vi "Create and Enqueue Self Launch.vi"(8 "error in (no error)":errorcluster) -> (0 "error out":errorcluster, 3 "Internal-Launch":refnum<event-registration>)   [LabVIEW 2018, in "Scripting.lvlib" / "Actor.lvlib" / "Actor.lvclass"]
uses:
  Actor.lvclass
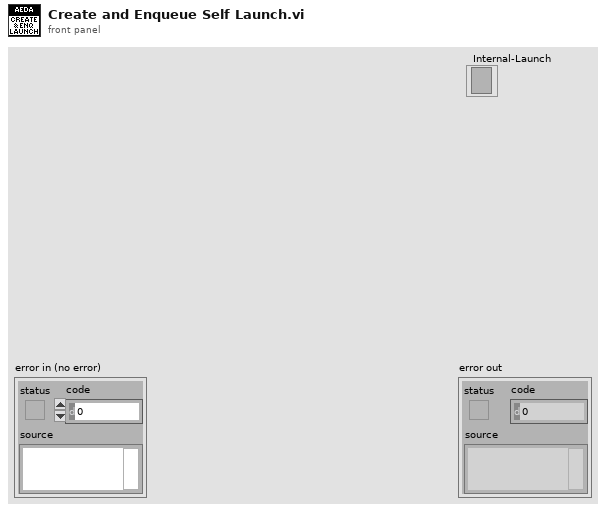
[diagram p1: front panel]
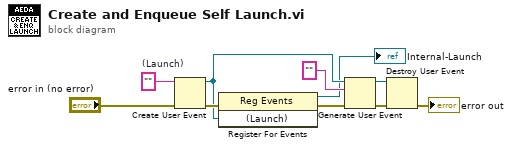
[diagram p0: block diagram]
diagram:
  w3 = ""  # (Launch)
  n1 = Create User Event(user event datatype=w3, error in="error in (no error)") -> (user event=w7:refnum<user-event>, error out=w10:errorcluster)
  n2 = register-events(error in=w10, w7) -> (reference out=→"Internal-Launch":refnum<event-registration>, error out=w8:errorcluster)  [unwired: 1 in]
  n3 = Generate User Event(user event=w7, event data cluster="" ("event data"), error in=w8) -> (user event out=w6:refnum<user-event>, error out=w5:errorcluster)  [unwired: 1 in]
  n4 = Destroy User Event(user event=w6, error in=w5) -> (error out=→"error out":errorcluster)
